vi "fgv_arboreal_parameters.vi"(7 "Function":T6, 8 "error in (no error)":errorcluster, 11 "Arboreal Scanning Parameters IN":T1={"Traced SWC file path"=path "", "Offsets"=[], "Scanning Type"=enum."Skeleton Scan", "Dwell Time"=0.1, "Segment Type"=enum."Fixed Length", "Length"=1.0, "Z fitting Wt."=1.0, "Fitting Threshold Mode"=enum."Max", "Finish Branches"=FALSE, "Length Limits"=[10.0, 1.0], "Frame Size"=200, "Fitting Threshold Score"=1000000000.0, "Field of View (mrad)"=0.0, "Display Options"=[FALSE, FALSE, FALSE, TRUE, TRUE], "Bounding Pixels"=5, "Relative Res."=1, "Field of View"=0.0, "XY Resampling"=1.0, "Z Resampling"=1.0, "Z Stack Info"=[]} {"Frame Size" items=["100X100"=100, "128X128"=128, "200X200"=200, "256X256"=256, "512X512"=512, "1024x1024"=1024, "2048x2048"=2048]}) -> (0 "error out":errorcluster, 3 "Arboreal Scanning Parameters OUT":T1={"Traced SWC file path"=path "", "Offsets"=[], "Scanning Type"=enum."Skeleton Scan", "Dwell Time"=0.1, "Segment Type"=enum."Fixed Length", "Length"=1.0, "Z fitting Wt."=1.0, "Fitting Threshold Mode"=enum."Max", "Finish Branches"=FALSE, "Length Limits"=[10.0, 1.0], "Frame Size"=200, "Fitting Threshold Score"=1000000000.0, "Field of View (mrad)"=0.0, "Display Options"=[FALSE, FALSE, FALSE, TRUE, TRUE], "Bounding Pixels"=5, "Relative Res."=1, "Field of View"=0.0, "XY Resampling"=1.0, "Z Resampling"=1.0, "Z Stack Info"=[]} {"Frame Size" items=["100X100"=100, "128X128"=128, "200X200"=200, "256X256"=256, "512X512"=512, "1024x1024"=1024, "2048x2048"=2048]})   [LabVIEW 2017]
uses:
  Typedefs/Read Write Enum.ctl
  Typedefs/Arboreal Scanning Parameters.ctl
  Typedefs/Arboreal Scan type.ctl
  Typedefs/Arboreal Segment Type.ctl
  Typedefs/Arboreal Fitting Threshold mode.ctl
  Typedefs/Frame Size.ctl
panel:
  # "Max Length"
  # "Min Length"
  # "(VL)"
  # "Max Length"
  # "Min Length"
  # "(VL)"
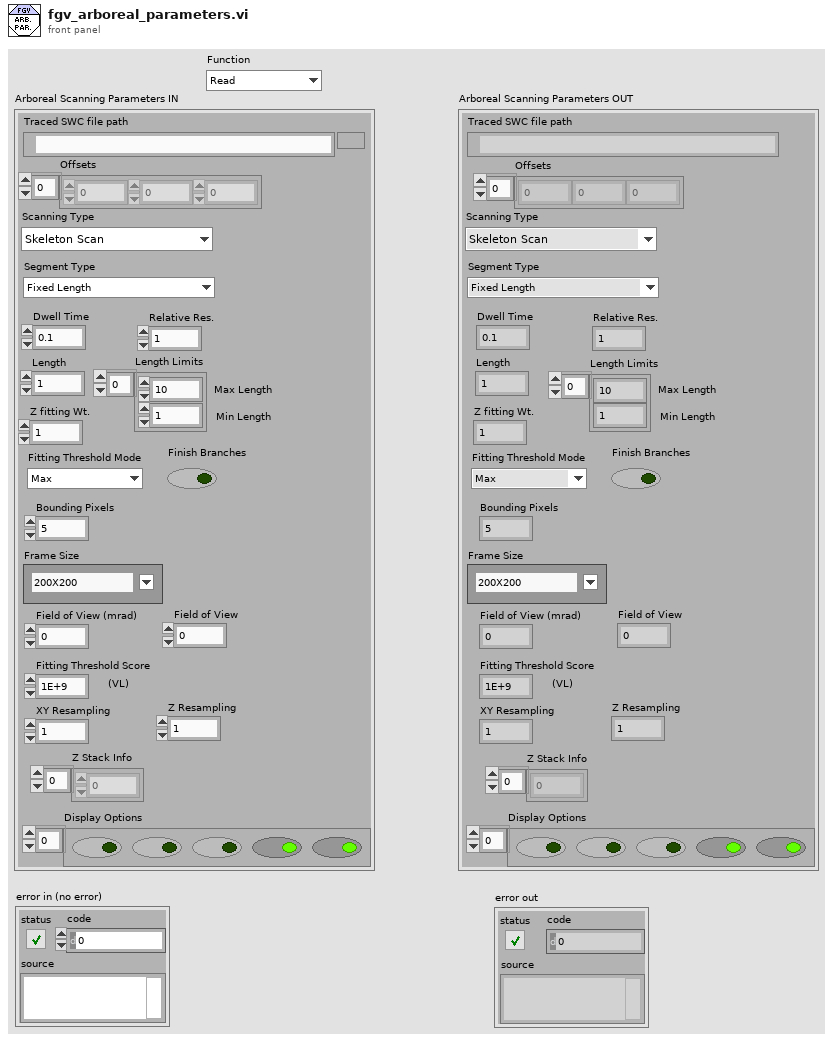
[diagram p1: front panel]
types:
  T1 = typedef "Arboreal Scanning Parameters.ctl" = cluster{"Traced SWC file path":path, "Offsets":dbl[], "Scanning Type":T2, "Dwell Time":dbl, "Segment Type":T3, "Length":dbl, "Z fitting Wt.":dbl, "Fitting Threshold Mode":T4, "Finish Branches":bool, "Length Limits":dbl[], "Frame Size":T5, "Fitting Threshold Score":dbl, "Field of View (mrad)":dbl, "Display Options":bool[], "Bounding Pixels":u16, "Relative Res.":u16, "Field of View":dbl, "XY Resampling":dbl, "Z Resampling":dbl, "Z Stack Info":dbl[]}
  T2 = typedef "Arboreal Scan type.ctl" = enum16{"Skeleton Scan", "Ribbon Scan", "Point Scan", "Buckshot Scan", "Mini Scan", "Volume Series Scan", "Volume Scan"}
  T3 = typedef "Arboreal Segment Type.ctl" = enum16{"Fixed Length", "Linear Fixed Length", "Variable Length", "Linear Variable Length", "2nd Order Polynomial", "3rd order Polynomial"}
  T4 = typedef "Arboreal Fitting Threshold mode.ctl" = enum16{"Max", "Median", "Mean"}
  T5 = typedef "Frame Size.ctl" = u16
  T6 = typedef "Read Write Enum.ctl" = enum16{"Read", "Write"}
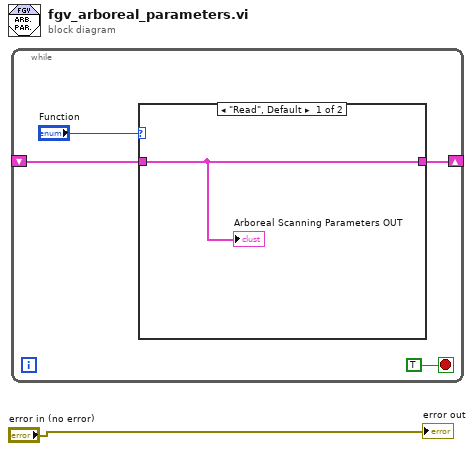
[diagram p0: block diagram]
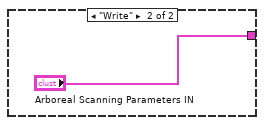
[diagram p2: hidden frame]
diagram:
  n1 = while {
    shift-right: [w5] -> _
    shift-left: _ -> [w4]
    stop <- TRUE stop-if-true
    n2 = case shown="\"Read\", Default" "Function" {
      tunnel: [w6 "Arboreal Scanning Parameters IN"] -> w5
      tunnel: w4 -> [w6 _]
      frame "Read", Default {
        "Arboreal Scanning Parameters OUT" <- w6
      }
      frame "Write" {
      }
    }
  }
  "error out" <- "error in (no error)"
